vi "Bridge_SCAN_USIDs.vi"(0 "HSDIO Sessions":T4, 1 "Potential_USID_Array":T1[](array[typedef])=[1, 2, 4, 7, 8, 9, 13, 15] max=15, 5 "Error In":errorcluster, 8 "Reg_Address_to_Read":T2={"First Reg Address"=31, "Num of Reg to Read"=1} {"Num of Reg to Read" min=1; "First Reg Address" format="%.0x"}) -> (14 "Registers_Readback":i32[](array[numeric]), 15 "USIDs_Detected":u8[](array[numeric]), 16 "Data_Readback":u8[](array[numeric])=[31, 144, 7], 18 "Converted Data":T3 {"Register" max=31 format="%.0x"; "Slave Address" max=15 format="%.0x"}, 19 "Error Out":errorcluster)   [LabVIEW 2013]
uses:
  Controls/USID.ctl
  Controls/Reg_Address_Data.ctl
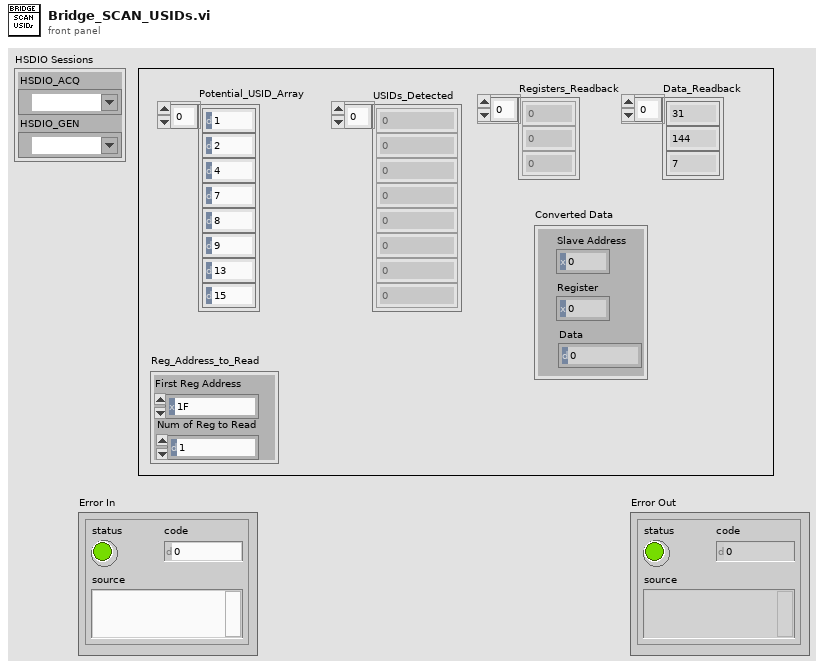
[diagram p1: front panel]
types:
  T1 = typedef "USID.ctl" = u8
  T2 = cluster{"First Reg Address":u8, "Num of Reg to Read":u8}
  T3 = cluster{"Slave Address":u8, "Register":u8, "Data":u8}
  T4 = cluster{"HSDIO_ACQ":refnum<k15>, "HSDIO_GEN":refnum<k15>}
  T5 = typedef "Reg_Address_Data.ctl" = cluster{"Address":u8, "Data":u8}
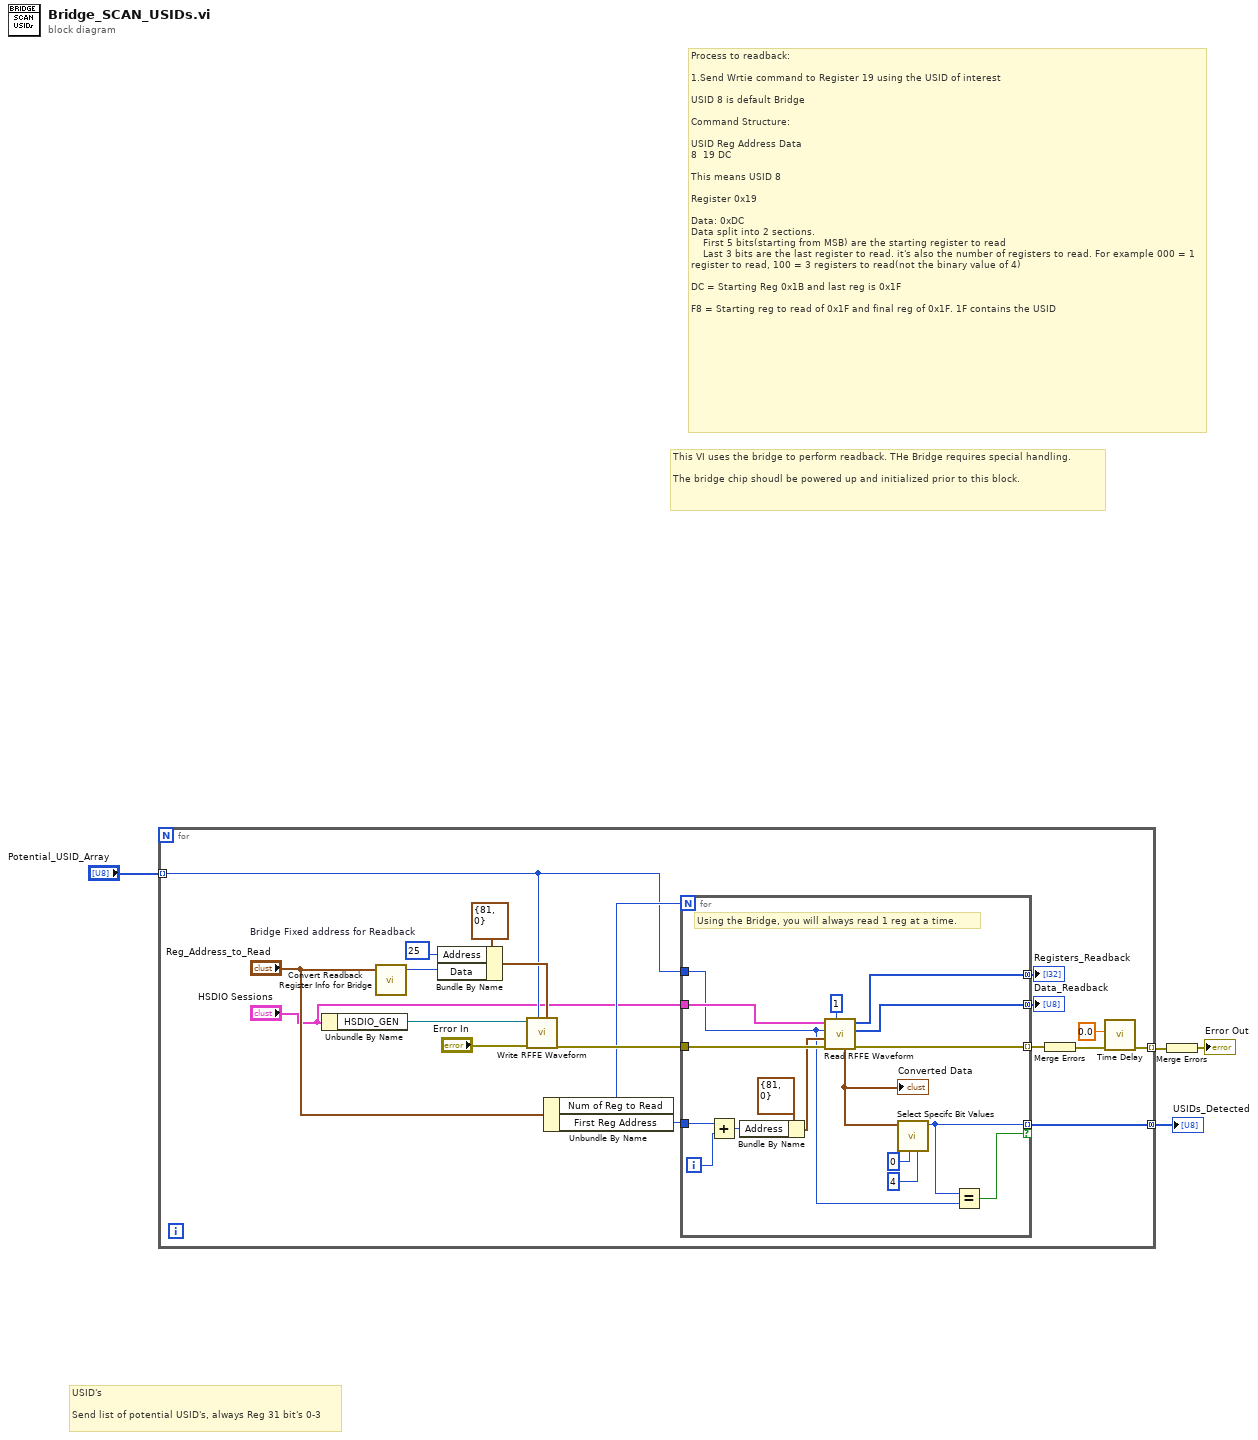
[diagram p0: block diagram]
diagram:
  # "USID's\n\nSend list of potential USID's, always Reg 31 bit's 0-3"
  # "Process to readback:\n\n1.Send Wrtie command to Register 19 using the USID of interest\n\nUSID 8 is default Bridge\n\nCommand Structure:\n\nUSID Reg Address Data\n8  19 DC\n\nThis means USID 8\n\nRegister 0x19\n\nData: 0xDC\nData split into 2 sections. \n    First 5 bits(starting from MSB) are the starting register to read\n    Last 3 bits are the last register to read. it's also the number of registers to read. For example 000 = 1 register to read, 100 = 3 registers to read(not the binary value of 4)\n\nDC = Starting Reg 0x1B and last reg is 0x1F\n\nF8 = Starting reg to read of 0x1F and final reg of 0x1F. 1F contains the USID"
  # "This VI uses the bridge to perform readback. THe Bridge requires special handling.\n\nThe bridge chip shoudl be powered up and initialized prior to this block."
  n1 = for {
    tunnel: "Potential_USID_Array" -> [w11] mode=indexing
    tunnel: [w10] -> w3 mode=concatenating
    tunnel: [w6] -> w2 mode=indexing
    w20 = u8 25  # Bridge Fixed address for Readback
    n2 = Unbundle By Name("HSDIO Sessions") -> ("HSDIO_GEN"=w12:refnum<k15>)
    n3 = call "Convert Readback Register Info for Bridge.vi"("Reg_Address_to_Read"="Reg_Address_to_Read") -> ("number"=w13:u32)  [unwired: 4 in]
    n4 = Bundle By Name(cluster=T5 {"Address"=81, "Data"=0} ("Reg_Address_Data"), "Address"=w20, "Data"=w13) -> (w19:T5)
    n5 = call "Write RFFE Waveform.vi"("Reg_Address_Data"=w19, "USID"=w11, "error in (no error)"="Error In", "instrument handle"=w12) -> ("error out"=w23:errorcluster)  [unwired: 5 in, 2 out]
    n6 = Unbundle By Name("Reg_Address_to_Read") -> ("Num of Reg to Read"=w15:u8, "First Reg Address"=w18:u8)
    n7 = for {
      N: w15 -> [_]
      tunnel: w23 -> [w40]
      tunnel: "HSDIO Sessions" -> [w39]
      tunnel: w11 -> [w27]
      tunnel: w18 -> [w33]
      tunnel: [w30] -> w17 mode=concatenating
      tunnel: [w29] -> w16 mode=concatenating
      tunnel: [w26] -> w10 mode=indexing if=w25
      tunnel: [w24] -> w8 mode=indexing
      i -> [w32]
      # "Using the Bridge, you will always read 1 reg at a time."
      n8 = Add(x=w33, y=w32) -> (x+y=w31:i32)
      n9 = Bundle By Name(cluster=T5 {"Address"=81, "Data"=0} ("Reg_Address_Data"), "Address"=w31) -> (w34:T5)
      n10 = call "Read RFFE Waveform.vi"("Number of Registers to Read"=u8 1, "error in (no error)"=w40, "Reg_Address_Data"=w34, "USID"=w27, "HSDIO Sessions"=w39) -> ("error out"=w24:errorcluster, "Ext_Read_Data"=w29:u8[], "Ext_Read_Reg"=w30:i32[], "Converted Data"=w37:T3)  [unwired: 2 in, 1 out]
      "Converted Data" <- w37
      n11 = call "Select Specifc Bit Values.vi"("#ofBits"=u8 4, "Bit_Location(LSB)"=u8 0, "Converted Data"=w37) -> ("Bits"=w26:u8)  [unwired: 8 in]
      n12 = Equal?(x=w26, y=w27) -> (x = y?=w25:bool)
    }
    "Registers_Readback" <- w17
    "Data_Readback" <- w16
    n13 = Merge Errors(w8) -> (w7:errorcluster)
    n14 = call "Time Delay"("error in (no error)"=w7, "Delay Time (s)"=0.0) -> ("error out"=w6:errorcluster)  [unwired: 9 in]
  }
  "USIDs_Detected" <- w3
  n15 = Merge Errors(w2) -> (→"Error Out":errorcluster)
